vi "Scatter.vi"(4 "Properties":T1={"Marker"={"Style"=enum."Automatic", "Color"=2147483647, "Size"=nan}, "Line"={"Style"=enum."Automatic", "Color"=2147483647, "Width"=nan}, "Colormap"={"Map"=enum."Automatic", "Value Min"=nan, "Value Max"=nan, "Scaling"=enum."Default", "Reverse"=FALSE}, "Display"={"Alpha"=nan, "Z Order"=nan}} {"Line"."Color" items=["Automatic"=2147483647, "Black"=0, "White"=16777215, "Red"=16711680, "Green"=2263842, "Blue"=255, "Cyan"=65535, "Magenta"=16711935, "Yellow"=16776960]; "Marker"."Color" items=["Automatic"=2147483647, "Black"=0, "White"=16777215, "Red"=16711680, "Green"=2263842, "Blue"=255, "Cyan"=65535, "Magenta"=16711935, "Yellow"=16776960]}, 5 "Colormap Values":dbl[](array[numeric]), 6 "Legend Title":string, 7 "Areas":dbl[](array[numeric]), 8 "error in (no error)":errorcluster, 9 "Y Data":dbl[](array[numeric]), 10 "X Data":dbl[](array[numeric]), 11 "Plot ID":T11 format="%x") -> (0 "error out":errorcluster, 3 "Plot ID Out":T11 format="%x")   [LabVIEW 2013, in "Advanced Plotting Toolkit.lvlib"]
doc: "Make a scatter plot, in which the data points are represented by discrete markers. Markers may have data-specific areas and colors."
uses:
  Advanced Plotting Toolkit.lvlib
  typedefs/PlotID.ctl
  ScatterProperties.ctl
  properties/Marker.ctl
  properties/Marker_Style.ctl
  typedefs/PlotColor.ctl
  properties/Line.ctl
  properties/Line_Style.ctl
  properties/Colormap.ctl
  properties/Colormap_Map.ctl
  properties/Colormap_Scaling.ctl
  properties/Display.ctl
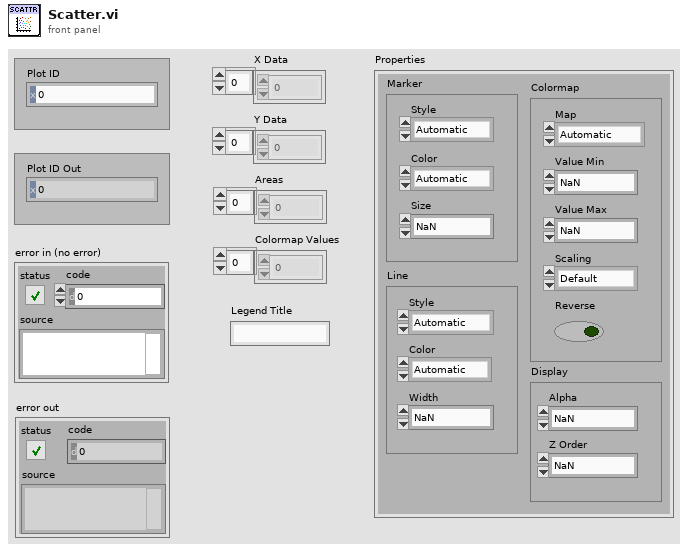
[diagram p1: front panel]
types:
  T1 = typedef "Advanced Plotting Toolkit.lvlib/ScatterProperties.ctl" = cluster{"Marker":T2, "Line":T5, "Colormap":T7, "Display":T10}
  T2 = typedef "Advanced Plotting Toolkit.lvlib/Marker.ctl" = cluster{"Style":T3, "Color":T4, "Size":dbl}
  T3 = typedef "Advanced Plotting Toolkit.lvlib/Marker_Style.ctl" = enum16{"Automatic", "Circle", "Square", "Triangle", "Diamond", "Star", "Invisible"}
  T4 = typedef "Advanced Plotting Toolkit.lvlib/PlotColor.ctl" = u32
  T5 = typedef "Advanced Plotting Toolkit.lvlib/Line.ctl" = cluster{"Style":T6, "Color":T4, "Width":sgl}
  T6 = typedef "Advanced Plotting Toolkit.lvlib/Line_Style.ctl" = enum16{"Automatic", "Solid", "Dashed", "Dotted", "Dash-dot", "Invisible"}
  T7 = typedef "Advanced Plotting Toolkit.lvlib/Colormap.ctl" = cluster{"Map":T8, "Value Min":dbl, "Value Max":dbl, "Scaling":T9, "Reverse":bool}
  T8 = typedef "Advanced Plotting Toolkit.lvlib/Colormap_Map.ctl" = enum16{"Automatic", "Rainbow", "Hot and Cold", "White-Black", "White-Blue", "White-Green", "White-Red", "Fire", "Water", "Earth", "Air", "Pastel", "Banded", "Stepped"}
  T9 = typedef "Advanced Plotting Toolkit.lvlib/Colormap_Scaling.ctl" = enum16{"Default"}
  T10 = typedef "Advanced Plotting Toolkit.lvlib/Display.ctl" = cluster{"Alpha":dbl, "Z Order":dbl}
  T11 = typedef "Advanced Plotting Toolkit.lvlib/PlotID.ctl" = i32
  T12 = typedef "Advanced Plotting Toolkit.lvlib/KeyValue.ctl" = cluster{"Key":string, "Value":string}
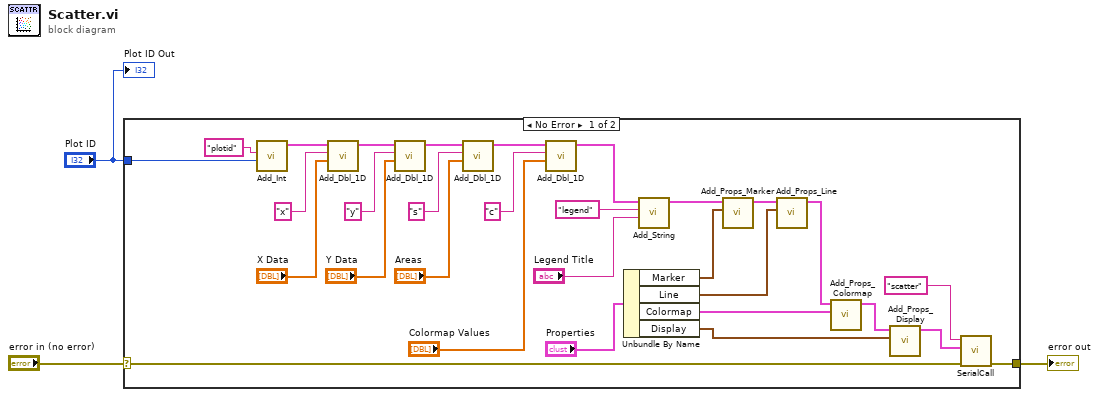
[diagram p0: block diagram]
diagram:
  n1 = case shown="No Error" "error in (no error)" {
    selector: "error in (no error)" -> [w17 w34]
    tunnel: "Plot ID" -> [w25 _]
    tunnel: [w16 w34] -> w1
    frame No Error {
      n2 = call "Add_Int.vi"("Value"=w25, "Key"="plotid") -> ("Keyword Array Out"=w23:T12[])  [unwired: 9 in]
      n3 = call "Add_Dbl_1D.vi"("Value"="X Data", "Key"="x", "Keyword Array"=w23) -> ("Keyword Array Out"=w22:T12[])  [unwired: 8 in]
      n4 = call "Add_Dbl_1D.vi"("Value"="Y Data", "Key"="y", "Keyword Array"=w22) -> ("Keyword Array Out"=w21:T12[])  [unwired: 8 in]
      n5 = call "Add_Dbl_1D.vi"("Value"="Areas", "Key"="s", "Keyword Array"=w21) -> ("Keyword Array Out"=w20:T12[])  [unwired: 8 in]
      n6 = call "Add_Dbl_1D.vi"("Value"="Colormap Values", "Key"="c", "Keyword Array"=w20) -> ("Keyword Array Out"=w7:T12[])  [unwired: 8 in]
      n7 = Unbundle By Name("Properties") -> ("Marker"=w13:T2, "Line"=w12:T5, "Colormap"=w11:T7, "Display"=w8:T10)
      n8 = call "Add_String.vi"("Value"="Legend Title", "Key"="legend", "Keyword Array"=w7) -> ("Keyword Array Out"=w6:T12[])  [unwired: 8 in]
      n9 = call "Add_Props_Marker.vi"("Marker"=w13, "Keyword Array"=w6) -> ("Keyword Array Out"=w15:T12[])  [unwired: 9 in]
      n10 = call "Add_Props_Line.vi"("Line"=w12, "Keyword Array"=w15) -> ("Keyword Array Out"=w19:T12[])  [unwired: 9 in]
      n11 = call "Add_Props_Colormap.vi"("Colormap"=w11, "Keyword Array"=w19) -> ("Keyword Array Out"=w10:T12[])  [unwired: 9 in]
      n12 = call "Add_Props_Display.vi"("Display"=w8, "Keyword Array"=w10) -> ("Keyword Array Out"=w9:T12[])  [unwired: 9 in]
      n13 = call "SerialCall.vi"("error in (no error)"=w17, "data"=w9, "Resource"="scatter") -> ("error out"=w16:errorcluster)  [unwired: 7 in, 1 out]
    }
    frame Error {
    }
  }
  "error out" <- w1
  "Plot ID Out" <- "Plot ID"
